vi "Initialize.vi"(11 "Zero Timeout Message Handler in":refnum<class "Zero Timeout Message Handler.lvclass">) -> (0 "error out":errorcluster, 3 "Zero Timeout Message Handler out":refnum<class "Zero Timeout Message Handler.lvclass">)   [LabVIEW 2024, in "Zero Timeout Message Handler.lvlib" / "Zero Timeout Message Handler.lvclass"]
uses:
  Zero Timeout Message Handler.lvclass
  Zero Timeout Message Handler.lvclass/Zero Timeout Message Handler.ctl
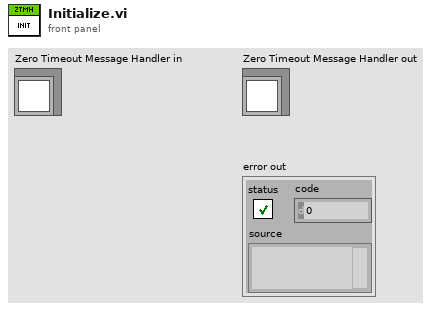
[diagram p1: front panel]
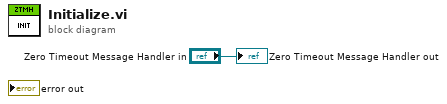
[diagram p0: block diagram]
diagram:
  "Zero Timeout Message Handler out" <- "Zero Timeout Message Handler in"
